vi "record_to_tsv.vi"(10 "cluster":cluster{"timestamp":timestamp, "value":dbl}, 11 "name":string) -> ()   [LabVIEW 2019]
uses:
  <vilib>/Utility/file.llb/Write Delimited Spreadsheet (string).vi
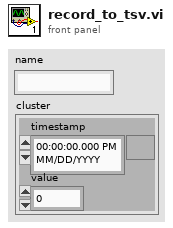
[diagram p1: front panel]
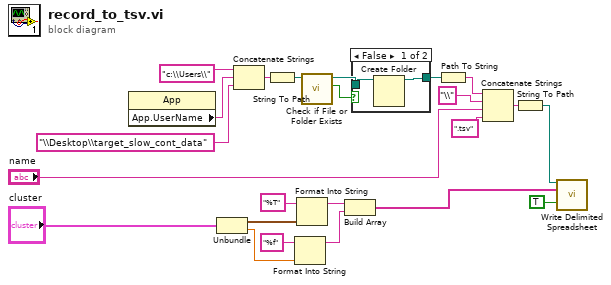
[diagram p0: block diagram]
diagram:
  w5 = "%T" ("format string")
  n1 = property class="App"() -> ("App.UserName"=w14:string)  [unwired: 2 in, 2 out]
  n2 = Unbundle("cluster") -> ("timestamp"=w23:timestamp, "value"=w21:dbl)
  n3 = Concatenate Strings("c:\\Users\\", w14, "\\Desktop\\target_slow_cont_data") -> (w12:string)
  n4 = String To Path(string=w12) -> (path=w7:path)
  n5 = Format Into String(format string="%f", w21) -> (resulting string=w18:string)  [unwired: 2 in, 1 out]
  n6 = Format Into String(format string=w5, initial string=w5, w23) -> (resulting string=w19:string)  [unwired: 1 in, 1 out]
  n7 = call <vilib>:"Check if File or Folder Exists.vi"("path"=w7) -> ("file or folder exists?"=w6:bool, "dup path"=w3:path)  [unwired: 8 in, 1 out]
  n8 = Build Array(w19, w18) -> (w17:string[])
  n9 = case shown="False" w6 {
    tunnel: w3 -> [w25 w26]
    tunnel: [w24 w26] -> w4
    frame False {
      n10 = Create Folder(path (use dialog)=w25) -> (created path=w24:path)  [unwired: 2 in, 2 out]
    }
    frame True {
    }
  }
  n11 = Path To String(path=w4) -> (string=w2:string)
  n12 = Concatenate Strings(w2, "\\", "name", ".tsv" ("string")) -> (w8:string)
  n13 = String To Path(string=w8) -> (path=w1:path)
  n14 = call-poly <vilib>:"Write Delimited Spreadsheet.vi"("file path (dialog if empty)"=w1, "1D data"=w17, "append to file? (new file:F)"=TRUE) -> ()  [unwired: 11 in, 2 out]
